vi "trace_display.vi"(0 "Carrier amplitudes":T13 format="%#_3p", 2 "Frequency display":T12, 3 "Spectrogram reference":refnum<vi>, 9 "Config":T19={"IO params"={"Conversion"={"Rate"=4.0, "Num cards"=2, "Out channels"=4}, "Carriers"={"Phase shift"=180.0, "Levels"=[[0.8, 0.8, 0.8], [0.03, 0.03, 0.03]], "Delay samples"=73.15}, "TCP"={"Host"="192.168.1.15", "Port"=6666, "Buffering"=6, "Timeout"=6}, "Input channel sign"=[1, 1, 1]}, "High rate STFT"={"Win param"=101.5, "Window type"=61, "Win order"=2, "DFT size"=64, "Channels"=[7], "Oversample"=64}, "Low rate STFT"={"Win param"=120.0, "Window type"=61, "Win order"=8, "DFT size"=64, "Channels"=[7], "Oversample"=64}, "Filtering "=[]} {"Filtering"."Distortion"."Limit" format="%#_3p"; "Filtering"."Distortion"."LF cut" format="%#_3p"; "Filtering"."Kalman"."Measure noise" format="%#_3p"; "Filtering"."Kalman"."Process noise" format="%#_3p"; "Filtering"."Hum"."Limit" format="%#_3p"; "Filtering"."Hum"."Frequency" format="%#_4p"; "Low rate STFT"."Oversample" min=1 step=1; "Low rate STFT"."Channels" min=0 step=1; "Low rate STFT"."DFT size" min=1 step=1; "Low rate STFT"."Window type" items=["Rectangle"=0, "Hanning"=1, "Hamming"=2, "Blackman-Harris"=3, "Exact Blackman"=4, "Blackman"=5, "Flat Top"=6, "4 Term B-Harris "=7, "7 Term B-Harris"=8, "Low Sidelobe"=9, "Blackman Nuttall"=11, "Triangle"=30, "Bartlett-Hanning"=31, "Bohman"=32, "Parzen"=33, "Welch"=34, "Kaiser"=60, "Dolph-Chebyshev"=61, "Gaussian"=62]; "High rate STFT"."Oversample" min=1 step=1; "High rate STFT"."Channels" min=0 step=1; "High rate STFT"."DFT size" min=1 step=1; "High rate STFT"."Window type" items=["Rectangle"=0, "Hanning"=1, "Hamming"=2, "Blackman-Harris"=3, "Exact Blackman"=4, "Blackman"=5, "Flat Top"=6, "4 Term B-Harris "=7, "7 Term B-Harris"=8, "Low Sidelobe"=9, "Blackman Nuttall"=11, "Triangle"=30, "Bartlett-Hanning"=31, "Bohman"=32, "Parzen"=33, "Welch"=34, "Kaiser"=60, "Dolph-Chebyshev"=61, "Gaussian"=62]; "IO params"."Input channel sign" min=-1 max=1 step=1; "IO params"."Carriers"."Levels" min=0.0 step=0.1; "IO params"."Conversion"."Rate" format="%#_8g"}, 10 "Reset":bool, 11 "Modulation info":T18 {"Hi channels at low" min=0 step=1; "Low carriers" format="%#_6p"; "High carriers" format="%#_6p"}, 12 "Display options":T3={"Display card"=0, "Signal"=enum."Raw data", "Source axis"=enum."X", "Sensor axis"=enum."X", "Spectrum parameters"={"Window"=enum."7 Term B-Harris", "FFT blocking"=enum."1", "Averaging"=5.0, "Order"=2}, "AC/DC"=FALSE, "Amplitude/Phase"=FALSE, "Levels selectors"=[], "Map selector"=enum."fire", "Restart Averaging"=FALSE, "Noise ref"=FALSE} {"Spectrum parameters"."Order" min=1 max=100; "Spectrum parameters"."Averaging" min=0.0 max=1000.0 step=1.0}, 13 "Trace info":T15) -> (20 "Autocorrelation":T1, 21 "Levels arrays":cluster{"Levels":dbl[][]}[](array[cluster]), 22 "STFT Spectrogram":dbl[][](array[numeric]), 23 "Time domain":waveform(dbl)[](array[waveform]), 24 "Time statistics":T14 {"dB" format="%.1f"; "RMS" format="%#_3p"; "DC" format="%#_3p"; "|max|" format="%#_3p"}, 25 "Spectrum":waveform(dbl)[](array[waveform]), 26 "Noise":T2 {"Noise delta" format="%#_6p"; "Noise floor" format="%#_6p"})   [LabVIEW 2026]
uses:
  processing/ilemt_config.ctl
  system/IO_params.ctl
  processing/stft_params.ctl
  <vilib>/Analysis/4window.llb/windowTd.ctl
  processing/filter_params.ctl
  processing/detrend_mode.ctl
  processing/modulation_info.ctl
  trace_info.ctl
  trace_channel.ctl
  main/ilemt_status.ctl
  trace_stats.ctl
  processing/carrier_amplitudes.ctl
  frequency_display_tabs.ctl
  display_options.ctl
  display_source.ctl
  axis_name.ctl
  spectrum_parameters.ctl
  levels_selector.ctl
  Level selector 1.ctl
  Level selector 4.ctl
  Level selector 3.ctl
  Level selector 2.ctl
  <vilib>/Analysis/2dsp.llb/1D Auto Correlation (DBL).vi
  main/ilemt_globals.vi
  <vilib>/Analysis/NI_AALPro.lvlib
panel:
  in  "Autocorrelation normalization":enum32{"none", "unbiased", "biased"}(ring)=enum."biased"
  # "Options:"
  # "High"
  # "Low"
  # "X"
  # "Y"
  # "Z"
  # "High"
  # "Low"
  # "X"
  # "Y"
  # "Z"
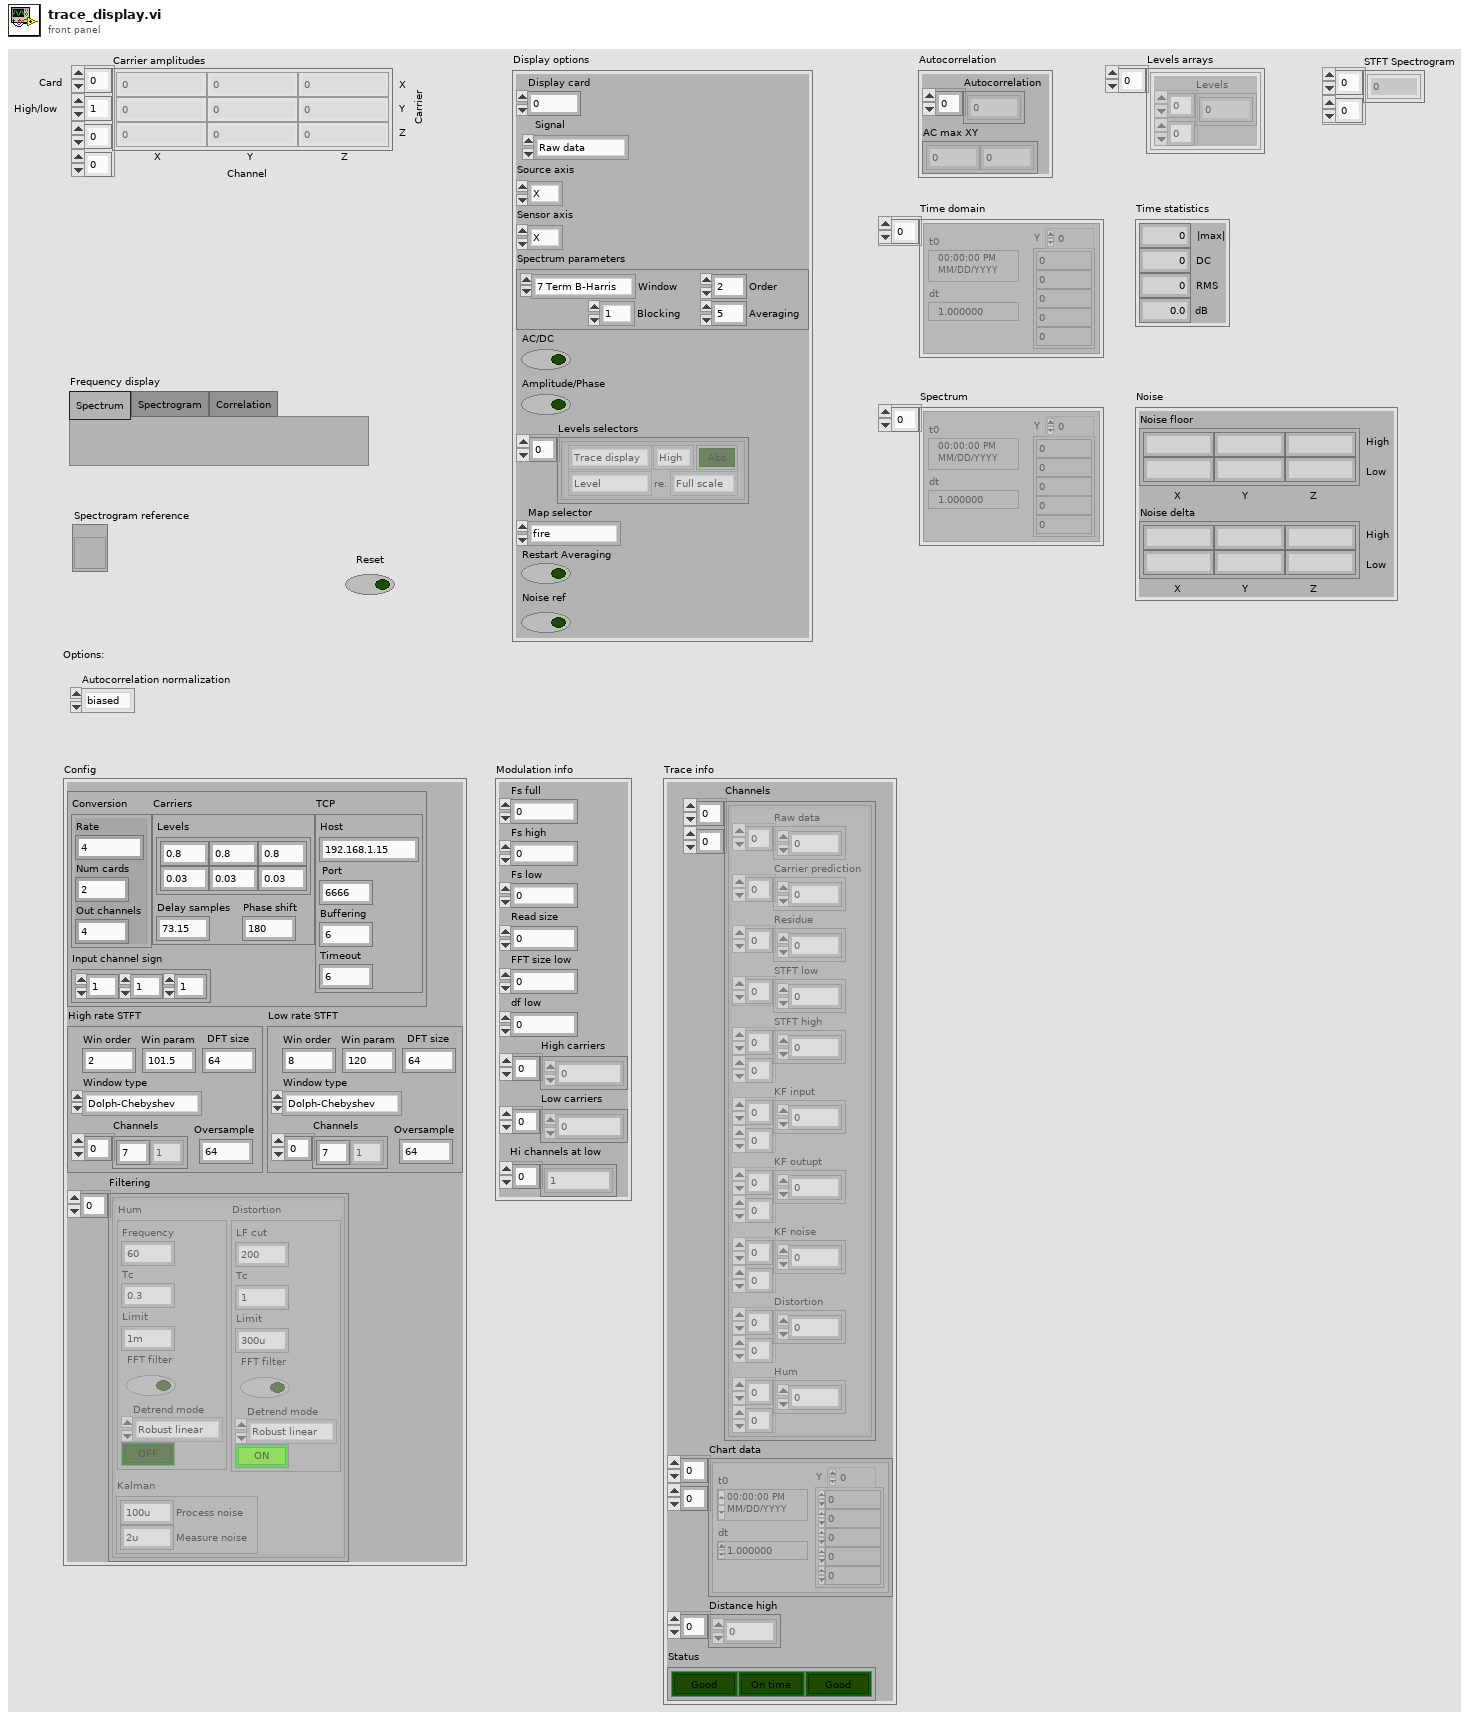
[diagram p1: front panel]
types:
  T1 = cluster{"Autocorrelation":dbl[], "AC max XY":dbl[]}
  T2 = cluster{"Noise floor":dbl[][], "Noise delta":dbl[][]}
  T3 = typedef "display_options.ctl" = cluster{"Display card":i32, "Signal":T4, "Source axis":T5, "Sensor axis":T5, "Spectrum parameters":T6, "AC/DC":bool, "Amplitude/Phase":bool, "Levels selectors":T7[], "Map selector":enum16{"fire", "rainbow", "grey", "inverse grey", "ice", "original"}, "Restart Averaging":bool, "Noise ref":bool}
  T4 = typedef "display_source.ctl" = enum16{"Raw data", "Carrier predict", "Residue", "STFT low", "STFT high", "KF input", "KF output", "KF noise", "Distortion", "Hum", "Distance high", "Chart high", "Chart low"}
  T5 = typedef "axis_name.ctl" = enum16{"X", "Y", "Z"}
  T6 = typedef "spectrum_parameters.ctl" = cluster{"Window":enum16{"None ", "Hanning", "Hamming", "Blackman-Harris", "Exact Blackman", "Blackman", "Flat Top", "4 Term B-Harris ", "7 Term B-Harris", "Low Sidelobe"}, "FFT blocking":enum16{"1", "2", "4", "8"}, "Averaging":dbl, "Order":u32}
  T7 = typedef "levels_selector.ctl" = cluster{"Signal source":T8, "Mode":T9, "re.":T10, "High/low":T11, "Sense":bool}
  T8 = typedef "Level selector 1.ctl" = enum16{"Trace display", "Carrier levels", "Ref levels"}
  T9 = typedef "Level selector 4.ctl" = enum16{"Level", "dB", "Phase", "Mismatch"}
  T10 = typedef "Level selector 3.ctl" = enum16{"Full scale", "Carrier", "Ref level", "Noise"}
  T11 = typedef "Level selector 2.ctl" = enum16{"High", "Low"}
  T12 = typedef "frequency_display_tabs.ctl" = enum32{"Spectrum", "Spectrogram", "Correlation"}
  T13 = typedef "carrier_amplitudes.ctl" = cdb[][][][]
  T14 = typedef "trace_stats.ctl" = cluster{"|max|":dbl, "DC":dbl, "RMS":dbl, "dB":dbl}
  T15 = typedef "trace_info.ctl" = cluster{"Channels":T16[][], "Chart data":waveform(dbl)[][], "Distance high":dbl[], "Status":T17}
  T16 = typedef "trace_channel.ctl" = cluster{"Raw data":dbl[], "Carrier prediction":dbl[], "Residue":dbl[], "STFT low":cdb[], "STFT high":cdb[][], "KF input":cdb[][], "KF outupt":cdb[][], "KF noise":dbl[][], "Distortion":cdb[][], "Hum":cdb[][]}
  T17 = typedef "ilemt_status.ctl" = cluster{"NaN":bool, "Backlog":bool, "Clipping":bool}
  T18 = typedef "modulation_info.ctl" = cluster{"Fs full":dbl, "Fs high":dbl, "Fs low":dbl, "Read size":i32, "FFT size low":i32, "df low":dbl, "High carriers":dbl[], "Low carriers":dbl[], "Hi channels at low":i32[]}
  T19 = typedef "ilemt_config.ctl" = cluster{"IO params":T20, "High rate STFT":T21, "Low rate STFT":T21, "Filtering ":T23[]}
  T20 = typedef "IO_params.ctl" = cluster{"Conversion":cluster{"Rate":dbl, "Num cards":u32, "Out channels":u32}, "Carriers":cluster{"Phase shift":dbl, "Levels":dbl[][], "Delay samples":dbl}, "TCP":cluster{"Host":string, "Port":i32, "Buffering":u32, "Timeout":u32}, "Input channel sign":i32[]}
  T21 = typedef "stft_params.ctl" = cluster{"Win param":dbl, "Window type":T22, "Win order":i32, "DFT size":i32, "Channels":i32[], "Oversample":i32}
  T22 = typedef "NI_AALPro.lvlib/windowTd.ctl" = u32
  T23 = typedef "filter_params.ctl" = cluster{"Hum":cluster{"Frequency":dbl, "Tc":dbl, "Limit":dbl, "FFT filter":bool, "Detrend mode":T24, "Enable":bool}, "Kalman":cluster{"Process noise":dbl, "Measure noise":dbl}, "Distortion":cluster{"LF cut":dbl, "Tc":dbl, "Limit":dbl, "FFT filter":bool, "Detrend mode":T24, "Enable":bool}}
  T24 = typedef "detrend_mode.ctl" = enum16{"Zero mean", "Linear", "Robust linear"}
  T25 = typedef "card_high_carrier_amplitudes.ctl" = cdb[][][]
  T26 = cluster{"Display card":i32, "Source axis":T5, "Signal":T4}
  T27 = enum16{"fire", "rainbow", "grey", "inverse grey", "ice", "original"}
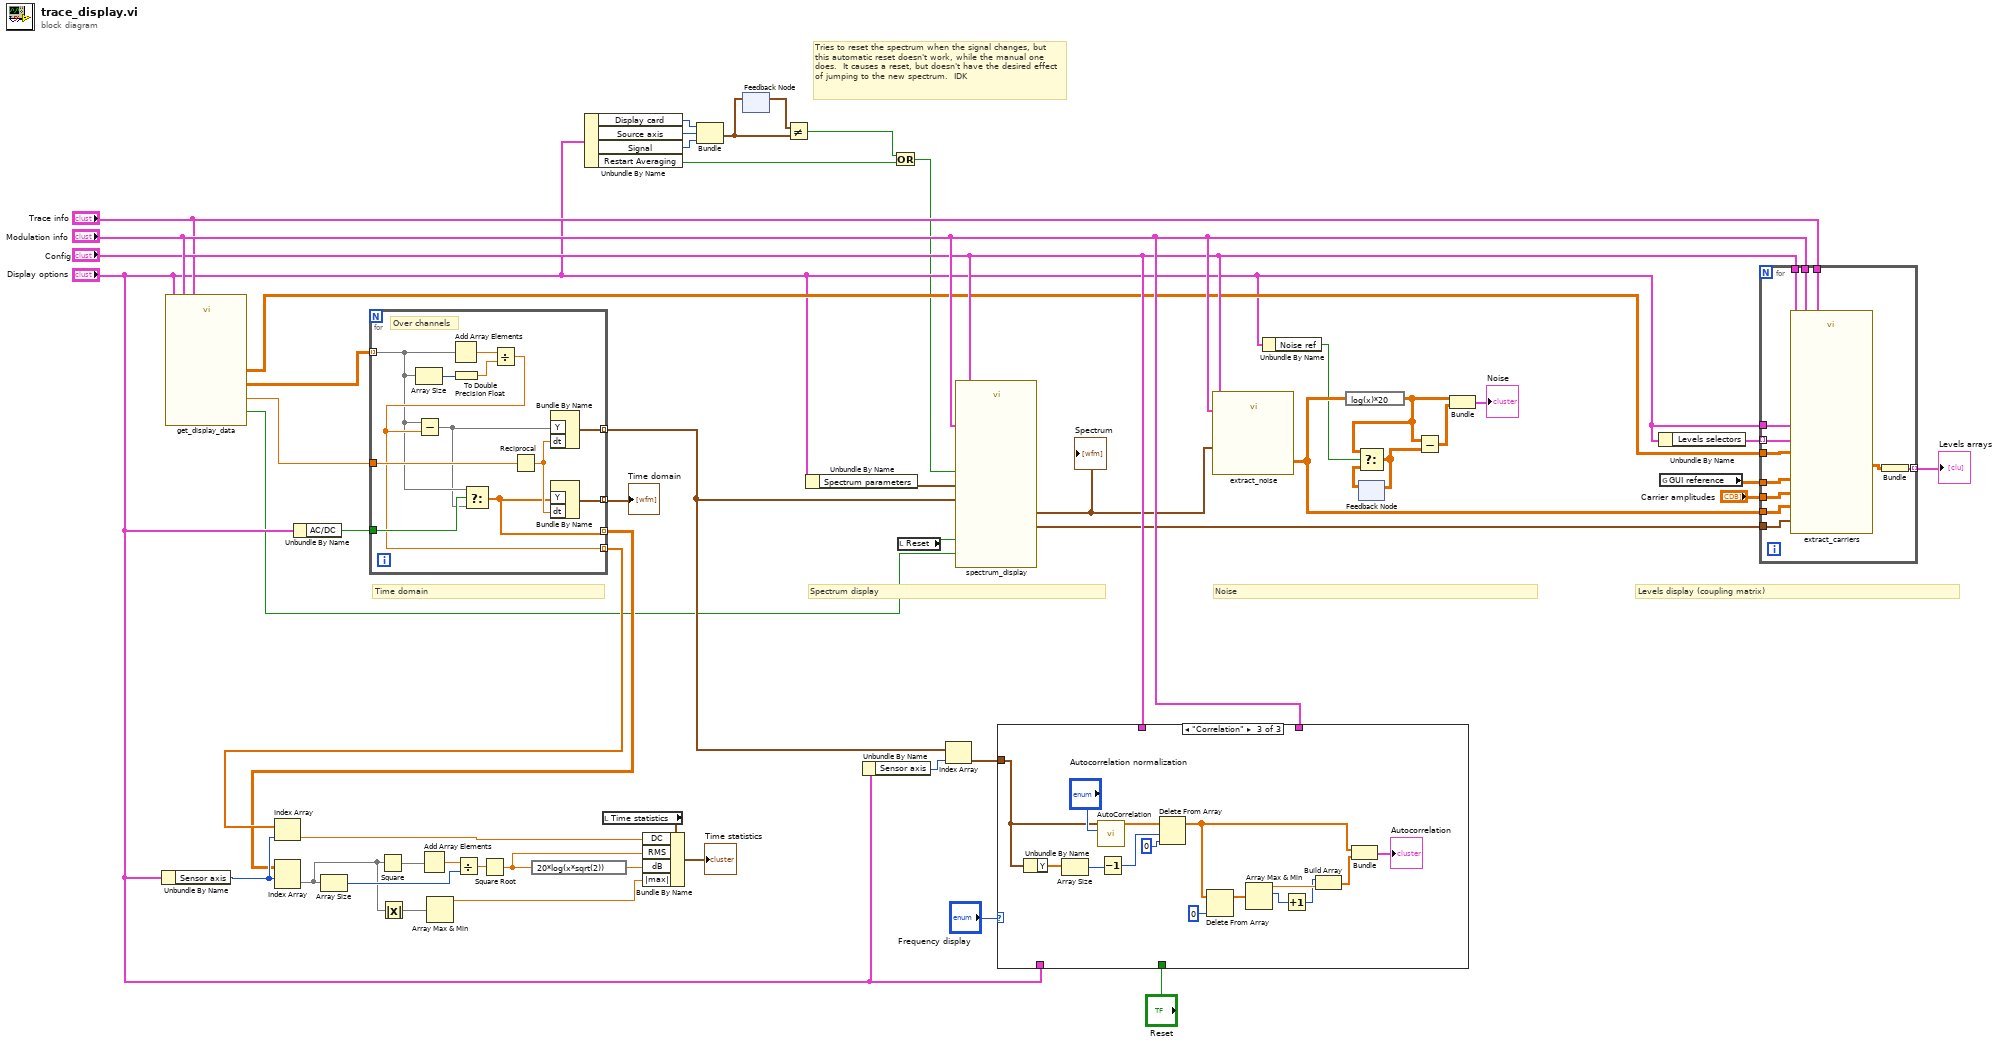
[diagram p0: block diagram]
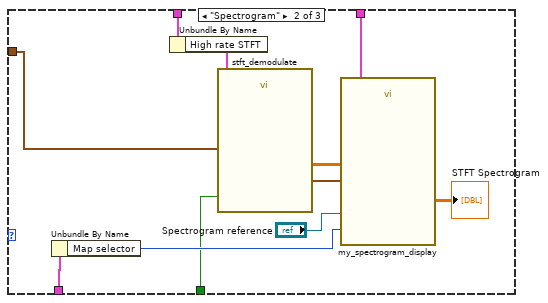
[diagram p3: hidden frame]
diagram:
  # "Tries to reset the spectrum when the signal changes, but this automatic reset doesn't work, while the manual one does.  It causes a reset, but doesn't have the desired effect of jumping to the new spectrum.  IDK"
  # "Time domain"
  # "Levels display (coupling matrix)"
  # "Noise"
  # "Spectrum display"
  n1 = Unbundle By Name("Display options") -> ("Sensor axis"=w22:T5)
  n2 = call "get_display_data.vi"("Modulation info"="Modulation info", "Trace info"="Trace info", "Display options"="Display options") -> ("Sample rate"=w15:dbl, "Demodulated signal"=w14:T25, "Time signal"=w38:dbl[][], "Chart data?"=w1:bool)  [unwired: 4 in, 1 out]
  n3 = Unbundle By Name("Display options") -> ("AC/DC"=w17:bool)
  n4 = for {
    tunnel: [w64] -> w41 mode=indexing
    tunnel: [w57] -> w40 mode=indexing
    tunnel: [w56] -> w20 mode=indexing
    tunnel: w15 -> [w61]
    tunnel: [w59] -> w13 mode=indexing
    tunnel: w38 -> [w55] mode=indexing
    tunnel: w17 -> [w58]
    # "Over channels"
    n5 = Array Size(array=w55) -> (size(s)=w65:i32)
    n6 = Add Array Elements(numeric array=w55) -> (sum=w63:dbl)
    n7 = To Double Precision Float(number=w65) -> (double precision float=w62:dbl)
    n8 = Divide(x=w63, y=w62) -> (x/y=w57:dbl)
    n9 = Subtract(x=w55, y=w57) -> (x-y=w54:dbl[])
    n10 = Select(t=w55, s=w58, f=w54) -> (s? t:f=w56:dbl[])
    n11 = Reciprocal(x=w61) -> (1/x=w60:dbl)
    n12 = Bundle By Name("Y"=w54, "dt"=w60) -> (w59:waveform(dbl))  [unwired: 1 in]
    n13 = Bundle By Name("Y"=w56, "dt"=w60) -> (w64:waveform(dbl))  [unwired: 1 in]
  }
  "Time domain" <- w41
  n14 = Index Array(array=w40, index=w22) -> (element=w39:dbl)
  n15 = Index Array(array=w20, index (row)=w22) -> (element=w35:dbl[])  [unwired: 1 in]
  n16 = Array Size(array=w35) -> (size(s)=w48:i32)
  n17 = Square(x=w35) -> (x^2=w51:dbl[])
  n18 = Absolute Value(x=w35) -> (abs(x)=w46:dbl[])
  n19 = Add Array Elements(numeric array=w51) -> (sum=w50:dbl)
  n20 = Array Max & Min(array=w46) -> (max value=w45:dbl)  [unwired: 3 out]
  n21 = Divide(x=w50, y=w48) -> (x/y=w49:dbl)
  n22 = Square Root(x=w49) -> (sqrt(x)=w42:dbl)
  n23 = expression code="20*log(x*sqrt(2))"(w42) -> (w43:dbl)
  n24 = Unbundle By Name("Display options") -> ("Display card"=w8:i32, "Source axis"=w10:T5, "Signal"=w9:T4, "Restart Averaging"=w4:bool)
  n25 = local read "Time statistics"() -> (w47:T14)
  n26 = Bundle By Name(cluster=w47, "DC"=w39, "RMS"=w42, "dB"=w43, "|max|"=w45) -> (→"Time statistics":T14)
  n27 = Bundle("Display card"=w8, "Source axis"=w10, "Signal"=w9) -> (w6:T26)  [unwired: 1 in]
  n28 = feedback #1() -> (w7:T26)  [unwired: 1 in]
  n29 = feedback-in #1(w6) -> ()
  n30 = Not Equal?(x=w7, y=w6) -> (x != y?=w3:bool)
  n31 = Unbundle By Name("Display options") -> ("Spectrum parameters"=w25:T6)
  n32 = Unbundle By Name("Display options") -> ("Sensor axis"=w21:T5)
  n33 = Or(x=w3, y=w4) -> (x .or. y?=w5:bool)
  n34 = local read "Reset"() -> (w2:bool)
  n35 = Index Array(array=w13, index=w21) -> (element=w19:waveform(dbl))
  n36 = call "spectrum_display.vi"("Chart data?"=w1, "Modulation info"="Modulation info", "Reset STFT"=w2, "Config"="Config", "Restart Averaging"=w5, "Spectrum parameters"=w25, "Time domain wavevorms"=w13) -> ("Complex spectrum"=w30:waveform(cdb)[], "dB spectrum"=w31:waveform(dbl)[])  [unwired: 3 in]
  "Spectrum" <- w31
  n37 = case shown="\"Correlation\"" "Frequency display" {
    tunnel: w19 -> [_ w71 w79]
    tunnel: "Config" -> [_ w70 _]
    tunnel: "Modulation info" -> [_ w69 _]
    tunnel: "Display options" -> [_ w68 _]
    tunnel: "Reset" -> [_ w66 _]
    frame "Spectrum", Default {
    }
    frame "Spectrogram" {
      n38 = Unbundle By Name(w68) -> ("Map selector"=w67:T27)
      n39 = Unbundle By Name(w70) -> ("High rate STFT"=w74:T21)
      n40 = call "stft_demodulate.vi"("STFT params"=w74, "Reset"=w66, "X"=w71) -> ("time-freq sample info"=w73:cluster{"time steps":i32, "frequency bins":i32}, "STFT"=w72:cdb[][])  [unwired: 6 in, 1 out]
      n41 = call "my_spectrogram_display.vi"("Modulation info"=w69, "time-freq sample info"=w73, "Map selector"=w67, "IntensityGraph in"="Spectrogram reference", "STFT {X}"=w72) -> ("STFT Spectrogram"=→"STFT Spectrogram":dbl[][])  [unwired: 6 in]
    }
    frame "Correlation" {
      n42 = Unbundle By Name(w79) -> ("Y"=w78:dbl[])
      n43 = Array Size(array=w78) -> (size(s)=w77:i32)
      n44 = call-poly <vilib>:"AutoCorrelation.vi"("normalization"="Autocorrelation normalization", "X"=w79) -> ("Rxx"=w83:dbl[])  [unwired: 8 in, 1 out]
      n45 = Decrement(x=w77) -> (x-1=w91:i32)
      n46 = Delete From Array(array=w83, length=w91, index=0) -> (array with subset deleted=w82:dbl[])  [unwired: 1 out]
      n47 = Delete From Array(array=w82, index=0) -> (array with subset deleted=w87:dbl[])  [unwired: 1 in, 1 out]
      n48 = Array Max & Min(array=w87) -> (max value=w86:dbl, max index (indices)=w85:i32)  [unwired: 2 out]
      n49 = Increment(x=w85) -> (x+1=w84:i32)
      n50 = Build Array(w84, w86) -> (w81:dbl[])
      n51 = Bundle("Rxx"=w82, w81) -> (→"Autocorrelation":cluster{"Rxx":dbl[], dbl[]})  [unwired: 1 in]
    }
  }
  n52 = call "extract_noise.vi"("Config"="Config", "Modulation info"="Modulation info", "Spectrum"=w31) -> ("Noise floor"=w34:dbl[][])  [unwired: 8 in]
  n53 = Unbundle By Name("Display options") -> ("Noise ref"=w29:bool)
  n54 = expression code="log(x)*20"(w34) -> (w28:dbl[][])
  n55 = feedback #2() -> (w33:dbl[][])  [unwired: 1 in]
  n56 = Select(t=w28, s=w29, f=w33) -> (s? t:f=w32:dbl[][])
  n57 = feedback-in #2(w32) -> ()
  n58 = Subtract(x=w28, y=w32) -> (x-y=w27:dbl[][])
  n59 = Bundle("Noise floor"=w28, w27) -> (→"Noise":cluster{"Noise floor":dbl[][], dbl[][]})  [unwired: 1 in]
  n60 = Unbundle By Name("Display options") -> ("Levels selectors"=w24:T7[])
  n61 = global read "ilemt_globals.vi" "GUI reference"() -> (w12:T13)
  n62 = for {
    tunnel: w30 -> [w103]
    tunnel: "Modulation info" -> [w102]
    tunnel: "Config" -> [w101]
    tunnel: w24 -> [w100] mode=indexing
    tunnel: [w98] -> w37 mode=indexing
    tunnel: w34 -> [w97]
    tunnel: "Trace info" -> [w96]
    tunnel: w12 -> [w95]
    tunnel: "Carrier amplitudes" -> [w94]
    tunnel: "Display options" -> [w93]
    tunnel: w14 -> [w92]
    n63 = call "extract_carriers.vi"("Carrier amplitudes"=w94, "Config"=w101, "Modulation info"=w102, "Demodulated signal"=w92, "Ref carrier amplitudes"=w95, "Display options"=w93, "Level selector"=w100, "Spectrum"=w103, "Trace info"=w96, "Noise floor"=w97) -> ("Levels"=w99:dbl[][])  [unwired: 9 in]
    n64 = Bundle("Levels"=w99) -> (w98:cluster{"Levels":dbl[][]})  [unwired: 1 in]
  }
  "Levels arrays" <- w37
